vi "Save Load Session.vi"(9 "Write":bool, 10 "Numeric Array In":dbl[](array[numeric]), 11 "Str Array in":string[](array[string])) -> (2 "Numeric Array Out":dbl[](array[numeric]), 3 "Str Array out":string[](array[string]))   [LabVIEW 2021]
uses:
  <vilib>/Utility/config.llb/Write Key (String).vi
  <vilib>/Utility/config.llb/Write Key (Double).vi
  <vilib>/Utility/config.llb/Read Key (String).vi
  <vilib>/Utility/config.llb/Read Key (Double).vi
  <vilib>/Utility/config.llb/NI_LVConfig.lvlib
panel:
  out "error out":errorcluster
  in  "error in (no error)":errorcluster
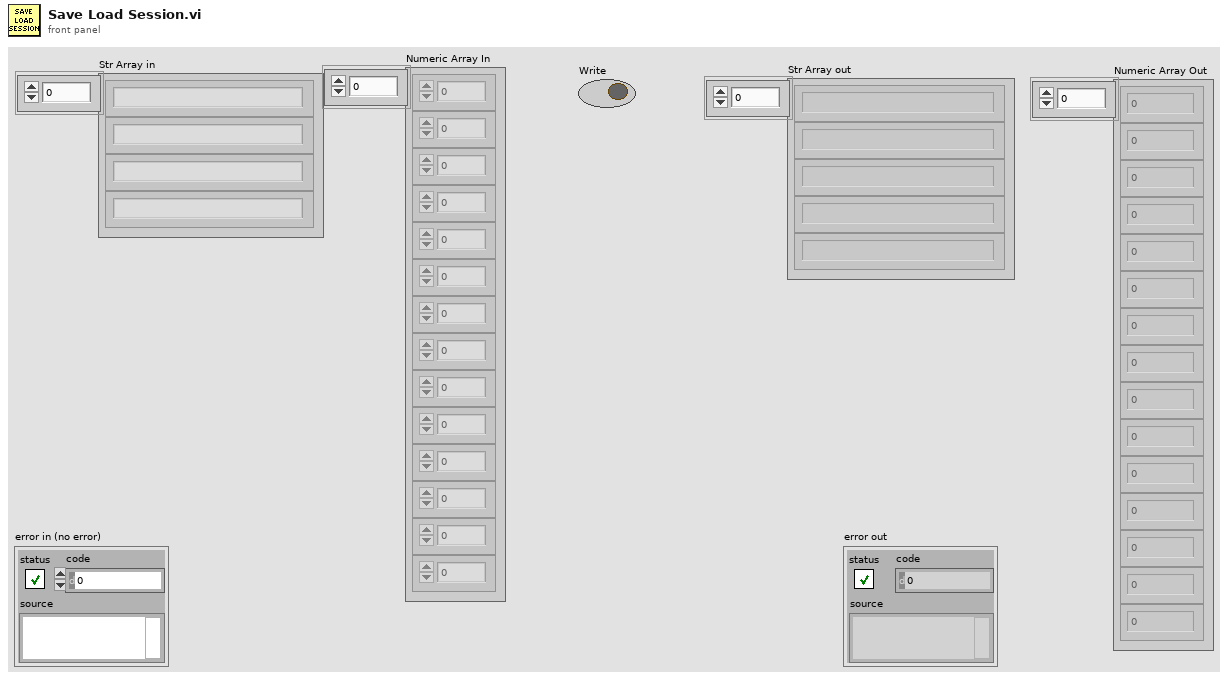
[diagram p1: front panel]
types:
  T1 = typedef "NI_LVConfig.lvlib/Config Data RefNum.ctl" = refnum<k1>
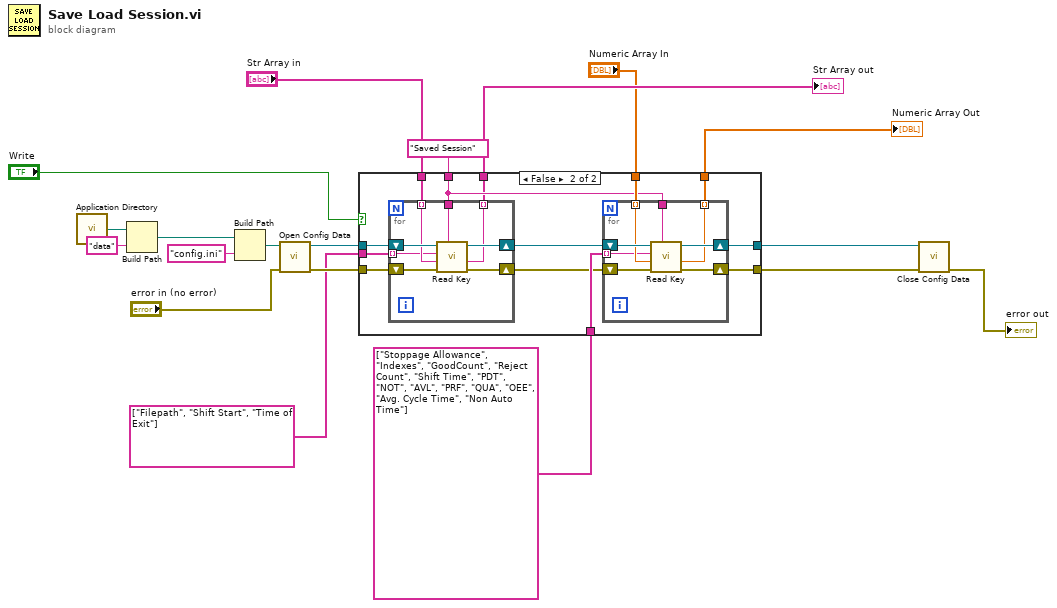
[diagram p0: block diagram]
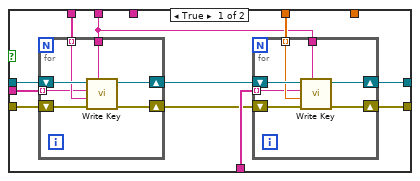
[diagram p2: hidden frame]
diagram:
  n1 = call <vilib>:"Application Directory.vi"() -> ("Application Directory"=w4:path)
  n2 = Build Path(base path=w4, name or relative path="data") -> (appended path=w6:path)
  n3 = Build Path(base path=w6, name or relative path="config.ini") -> (appended path=w15:path)
  n4 = call <vilib>:"Open Config Data.vi"("error in (no error)"="error in (no error)", "configuration file path"=w15) -> ("error out"=w12:errorcluster, "refnum"=w11:T1)  [unwired: 7 in, 1 out]
  n5 = case shown="False" "Write" {
    tunnel: string[] ["Stoppage Allowance", "Indexes", "GoodCount", "Reject Count", "Shift Time", "PDT", "NOT", "AVL", "PRF", "QUA", "OEE", "Avg. Cycle Time", "Non Auto Time"] -> [w30 w57]
    tunnel: "Numeric Array In" -> [w29 w56]
    tunnel: string[] ["Filepath", "Shift Start", "Time of Exit"] -> [w26 w53]
    tunnel: "Str Array in" -> [w25 w47]
    tunnel: w11 -> [w24 w52]
    tunnel: w12 -> [w23 w51]
    tunnel: [w22 w50] -> w13
    tunnel: [w21 w49] -> w14
    tunnel: "Saved Session" ("section") -> [w20 w48]
    tunnel: [_ w46] -> w18
    tunnel: [_ w45] -> w19
    frame True {
      n6 = for {
        tunnel: w20 -> [w35]
        shift-right: [w37] -> w27
        shift-left: w24 -> [w34]
        shift-right: [w36] -> w28
        shift-left: w23 -> [w33]
        tunnel: w25 -> [w32] mode=indexing
        tunnel: w26 -> [w31] mode=indexing
        n7 = call-poly <vilib>:"Write Key.vi"("section"=w35, "error in (no error)"=w33, "value"=w32, "key"=w31, "refnum"=w34) -> ("error out"=w36:errorcluster, "refnum out"=w37:T1)  [unwired: 4 in, 1 out]
      }
      n8 = for {
        tunnel: w20 -> [w42]
        shift-right: [w44] -> w22
        shift-left: w27 -> [w41]
        shift-right: [w43] -> w21
        shift-left: w28 -> [w40]
        tunnel: w29 -> [w39] mode=indexing
        tunnel: w30 -> [w38] mode=indexing
        n9 = call-poly <vilib>:"Write Key.vi"("section"=w42, "error in (no error)"=w40, "value"=w39, "key"=w38, "refnum"=w41) -> ("error out"=w43:errorcluster, "refnum out"=w44:T1)  [unwired: 4 in, 1 out]
      }
    }
    frame False {
      n10 = for {
        tunnel: w48 -> [w63]
        shift-right: [w65] -> w54
        shift-left: w52 -> [w62]
        shift-right: [w64] -> w55
        shift-left: w51 -> [w61]
        tunnel: w47 -> [w60] mode=indexing
        tunnel: w53 -> [w59] mode=indexing
        tunnel: [w58] -> w46 mode=indexing
        n11 = call-poly <vilib>:"Read Key.vi"("section"=w63, "error in (no error)"=w61, "default value"=w60, "key"=w59, "refnum"=w62) -> ("error out"=w64:errorcluster, "value"=w58:string, "refnum out"=w65:T1)  [unwired: 3 in, 1 out]
      }
      n12 = for {
        tunnel: w48 -> [w71]
        shift-right: [w73] -> w50
        shift-left: w54 -> [w70]
        shift-right: [w72] -> w49
        shift-left: w55 -> [w69]
        tunnel: w56 -> [w68] mode=indexing
        tunnel: w57 -> [w67] mode=indexing
        tunnel: [w66] -> w45 mode=indexing
        n13 = call-poly <vilib>:"Read Key.vi"("section"=w71, "error in (no error)"=w69, "default value"=w68, "key"=w67, "refnum"=w70) -> ("error out"=w72:errorcluster, "value"=w66:dbl, "refnum out"=w73:T1)  [unwired: 3 in, 1 out]
      }
    }
  }
  "Numeric Array Out" <- w19
  "Str Array out" <- w18
  n14 = call <vilib>:"Close Config Data.vi"("error in (no error)"=w14, "refnum"=w13) -> ("error out"=→"error out":errorcluster)  [unwired: 8 in, 1 out]
